vi "getU16.vi"(7 "offset":i32, 8 "String":string) -> (3 "value":i32)   [LabVIEW 2013]
doc: "Get an U16 from string at offset"
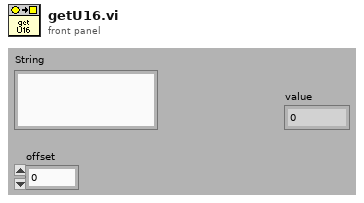
[diagram p1: front panel]
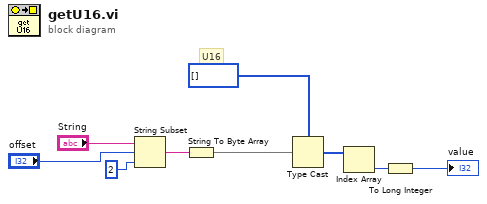
[diagram p0: block diagram]
diagram:
  # "U16"
  n1 = String Subset(string="String", offset (0)="offset", length (rest)=2 ("length (rest)")) -> (substring=w6:string)
  n2 = String To Byte Array(string=w6) -> (unsigned byte array=w1:u8[])
  n3 = Type Cast(type=u16[] [], x=w1) -> (*(type *) &x=w4:u16[])
  n4 = Index Array(array=w4) -> (element=w3:u16)  [unwired: 1 in]
  n5 = To Long Integer(number=w3) -> (32bit integer=→"value":i32)
